vi "A01423754_Ximena_Avila_Ejercicio_04_base_a_base_17_Enero_X(1).vi"() -> ()   [LabVIEW 2018]
panel:
  in  "Numero":string
  out "Nuevo numero":string
  in  "Nueva base":u64
  in  "Base":u64
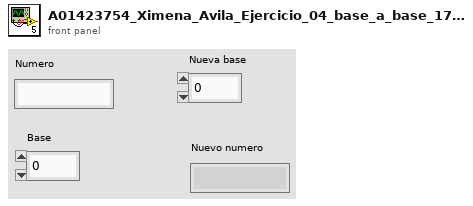
[diagram p1: front panel]
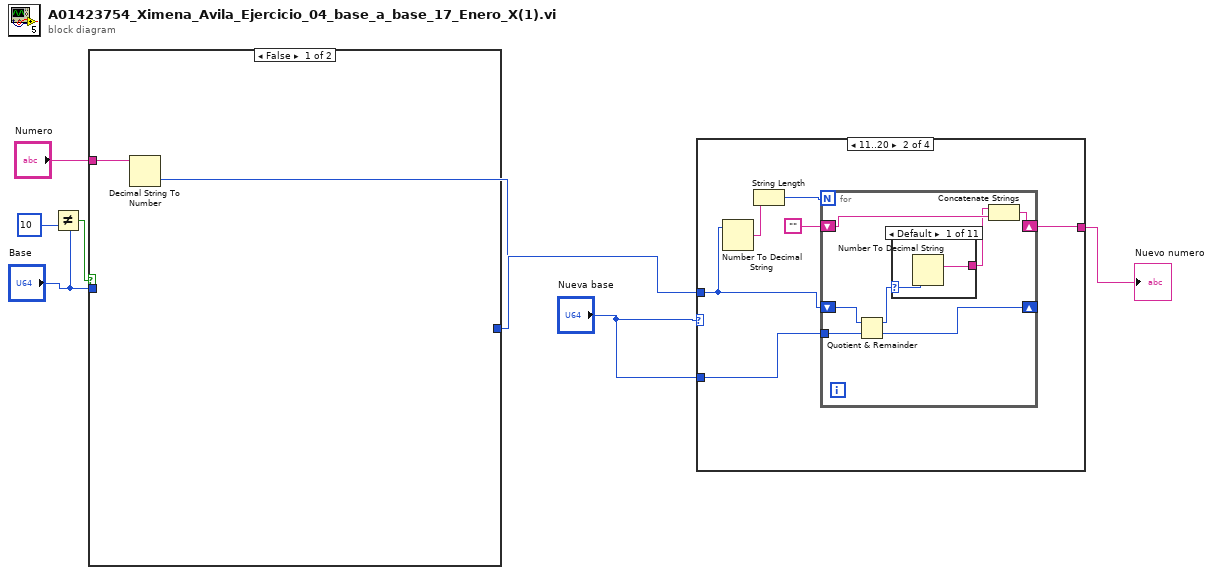
[diagram p0: block diagram]
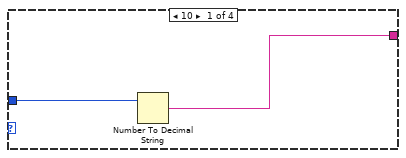
[diagram p2: hidden frame]
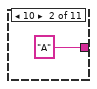
[diagram p3: hidden frame]
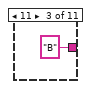
[diagram p4: hidden frame]
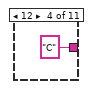
[diagram p5: hidden frame]
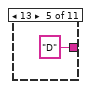
[diagram p6: hidden frame]
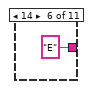
[diagram p7: hidden frame]
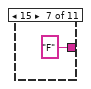
[diagram p8: hidden frame]
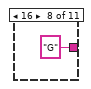
[diagram p9: hidden frame]
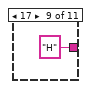
[diagram p10: hidden frame]
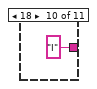
[diagram p11: hidden frame]
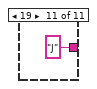
[diagram p12: hidden frame]
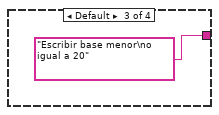
[diagram p13: hidden frame]
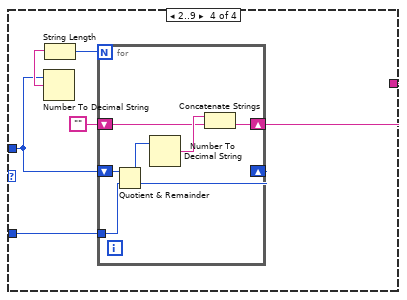
[diagram p14: hidden frame]
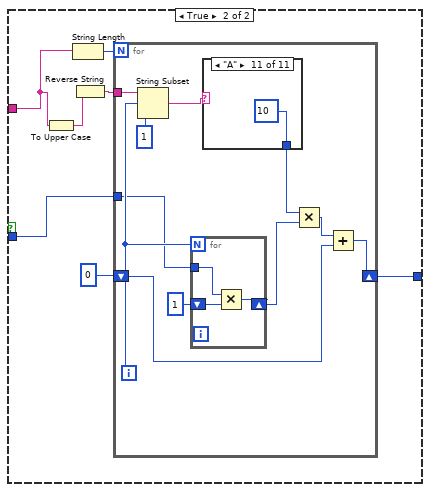
[diagram p15: hidden frame]
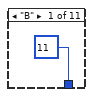
[diagram p16: hidden frame]
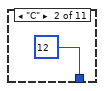
[diagram p17: hidden frame]
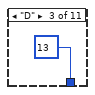
[diagram p18: hidden frame]
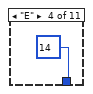
[diagram p19: hidden frame]
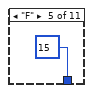
[diagram p20: hidden frame]
diagram:
  n1 = Not Equal?(x="Base", y=u64 10) -> (x != y?=w6:bool)
  n2 = case shown="False" w6 {
    tunnel: "Base" -> [_ w15]
    tunnel: [w8 w14] -> w3
    tunnel: "Numero" -> [w9 w10]
    frame False {
      n3 = Decimal String To Number(string=w9) -> (number=w8:i32)  [unwired: 2 in, 1 out]
    }
    frame True {
      n4 = To Upper Case(1:w10) -> (0:w11:string)
      n5 = String Length(string=w10) -> (length=w16:i32)
      n6 = Reverse String(1:w11) -> (0:w13:string)
      n7 = for {
        N: w16 -> [_]
        tunnel: w15 -> [w25]
        shift-right: [w22] -> w14
        shift-left: 0 -> [w21]
        tunnel: w13 -> [w19]
        i -> [w26]
        n8 = String Subset(string=w19, offset (0)=w26, length (rest)=1 ("length (rest)")) -> (substring=w18:string)
        n9 = for {
          N: w26 -> [_]
          tunnel: w25 -> [w42]
          shift-right: [w41] -> w24
          shift-left: u64 1 -> [w40]
          n10 = Multiply(x=w42, y=w40) -> (x*y=w41:u64)
        }
        n11 = case shown="\"A\"" w18 {
          selector: w18 -> [_ _ _ _ _ _ _ _ _ w37 _]
          tunnel: [11 12 13 14 15 16 17 18 19 w38 10] -> w17
          frame "B" {
          }
          frame "C" {
          }
          frame "D" {
          }
          frame "E" {
          }
          frame "F" {
          }
          frame "G" {
          }
          frame "H" {
          }
          frame "I" {
          }
          frame "J" {
          }
          frame Default {
            n12 = Decimal String To Number(string=w37) -> (number=w38:i32)  [unwired: 2 in, 1 out]
          }
          frame "A" {
          }
        }
        n13 = Multiply(x=w17, y=w24) -> (x*y=w23:u64)
        n14 = Add(x=w23, y=w21) -> (x+y=w22:u64)
      }
    }
  }
  n15 = case shown="11..20" "Nueva base" {
    tunnel: w3 -> [w44 w47 _ w74]
    tunnel: [w43 w45 "Escribir base menor\no igual a 20" w72] -> w4
    tunnel: "Nueva base" -> [_ w46 _ w71]
    frame 10 {
      n16 = Number To Decimal String(number=w44) -> (decimal integer string=w43:string)  [unwired: 1 in]
    }
    frame 11..20 {
      n17 = Number To Decimal String(number=w47) -> (decimal integer string=w50:string)  [unwired: 1 in]
      n18 = String Length(string=w50) -> (length=w49:i32)
      n19 = for {
        N: w49 -> [_]
        shift-right: [w53] -> w45
        shift-left: "" -> [w52]
        shift-right: [w56] -> _
        shift-left: w47 -> [w57]
        tunnel: w46 -> [w55]
        n20 = Quotient & Remainder(x=w57, y=w55) -> (x-y*floor(x/y)=w54:u64, floor(x/y)=w56:u64)
        n21 = case shown="Default" w54 {
          selector: w54 -> [w59 _ _ _ _ _ _ _ _ _ _]
          tunnel: [w58 "A" "B" "C" "D" "E" "F" "G" "H" "I" "J"] -> w51
          frame Default {
            n22 = Number To Decimal String(number=w59) -> (decimal integer string=w58:string)  [unwired: 1 in]
          }
          frame 10 {
          }
          frame 11 {
          }
          frame 12 {
          }
          frame 13 {
          }
          frame 14 {
          }
          frame 15 {
          }
          frame 16 {
          }
          frame 17 {
          }
          frame 18 {
          }
          frame 19 {
          }
        }
        n23 = Concatenate Strings(w51, w52) -> (w53:string)
      }
    }
    frame Default {
    }
    frame 2..9 {
      n24 = Number To Decimal String(number=w74) -> (decimal integer string=w76:string)  [unwired: 1 in]
      n25 = String Length(string=w76) -> (length=w75:i32)
      n26 = for {
        N: w75 -> [_]
        shift-right: [w77] -> _
        shift-left: w74 -> [w83]
        tunnel: w71 -> [w82]
        shift-right: [w79] -> w72
        shift-left: "" -> [w78]
        n27 = Quotient & Remainder(x=w83, y=w82) -> (x-y*floor(x/y)=w81:u64, floor(x/y)=w77:u64)
        n28 = Number To Decimal String(number=w81) -> (decimal integer string=w80:string)  [unwired: 1 in]
        n29 = Concatenate Strings(w80, w78) -> (w79:string)
      }
    }
  }
  "Nuevo numero" <- w4
